vi "Initialize Intermediate Buffers.vi"(8 "error in (no error)":errorcluster, 10 "largest block count":u64, 11 "Buffer Converter in":refnum<class "Buffer Converter.lvclass">) -> (0 "error out":errorcluster, 3 "Buffer Converter out":refnum<class "Buffer Converter.lvclass">)   [LabVIEW 2017, in "DSF Core.lvlib" / "Buffer Converter.lvclass"]
uses:
  Buffer Converter.lvclass
  Typedefs/DSF Runtime Type Buffers.ctl
  Buffer Converter.lvclass/Buffer Converter.ctl
  DSF Core.lvlib
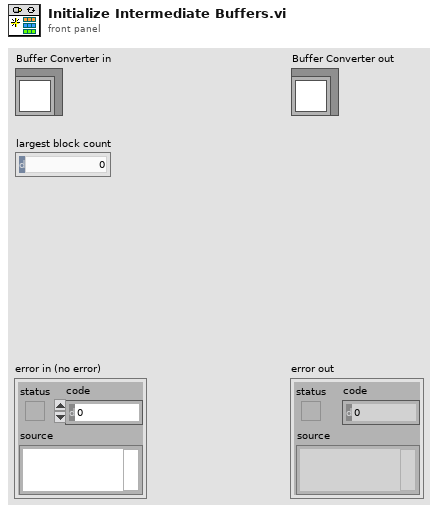
[diagram p1: front panel]
types:
  T1 = typedef "DSF Core.lvlib/DSF Runtime Type Buffers.ctl" = cluster{"Bool":bool[], "SGL":sgl[], "DBL":dbl[], "I8":i8[], "I16":i16[], "I32":i32[], "I64":i64[], "U8":u8[], "U16":u16[], "U32":u32[], "U64":u64[]}
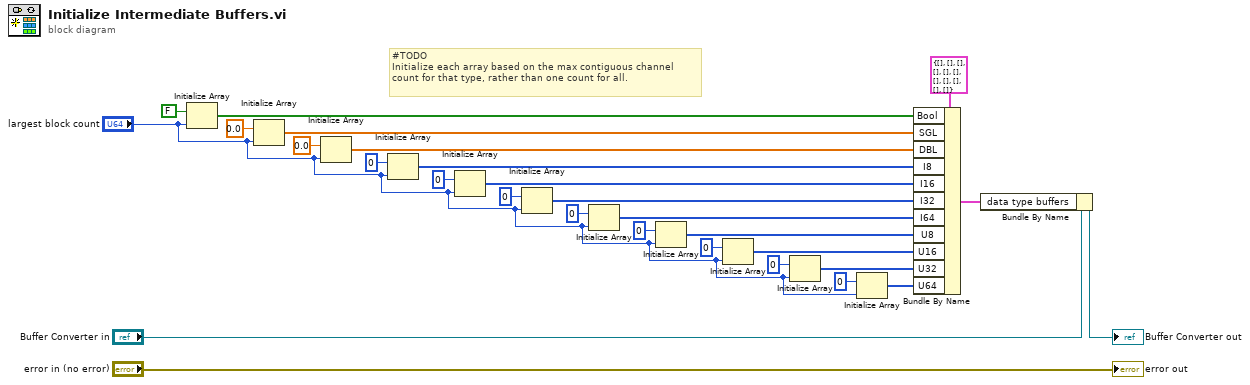
[diagram p0: block diagram]
diagram:
  # "#TODO\nInitialize each array based on the max contiguous channel count for that type, rather than one count for all."
  n1 = Initialize Array(FALSE, "largest block count") -> (w25:bool[])
  n2 = Initialize Array(sgl 0.0, "largest block count") -> (w24:sgl[])
  n3 = Initialize Array(0.0, "largest block count") -> (w21:dbl[])
  n4 = Initialize Array(i8 0, "largest block count") -> (w6:i8[])
  n5 = Initialize Array(i16 0, "largest block count") -> (w7:i16[])
  n6 = Initialize Array(0, "largest block count") -> (w8:i32[])
  n7 = Initialize Array(i64 0, "largest block count") -> (w9:i64[])
  n8 = Initialize Array(u8 0, "largest block count") -> (w10:u8[])
  n9 = Initialize Array(u16 0, "largest block count") -> (w11:u16[])
  n10 = Initialize Array(u32 0, "largest block count") -> (w12:u32[])
  n11 = Initialize Array(u64 0, "largest block count") -> (w13:u64[])
  n12 = Bundle By Name(cluster=T1 {"Bool"=[], "SGL"=[], "DBL"=[], "I8"=[], "I16"=[], "I32"=[], "I64"=[], "U8"=[], "U16"=[], "U32"=[], "U64"=[]} ("Data Type Buffers"), "Bool"=w25, "SGL"=w24, "DBL"=w21, "I8"=w6, "I16"=w7, "I32"=w8, "I64"=w9, "U8"=w10, "U16"=w11, "U32"=w12, "U64"=w13) -> (w2:T1)
  n13 = Bundle By Name(cluster="Buffer Converter in", "data type buffers"=w2) -> (→"Buffer Converter out":refnum<class "Buffer Converter.lvclass">)
  "error out" <- "error in (no error)"
